vi "XY Graph Get Plot Name Format String.vi"(8 "error in (no error)":errorcluster, 11 "Select(T)/Deselect(F)":bool) -> (0 "error out":errorcluster, 1 "Cancelled?":bool, 3 "String Format":string)   [LabVIEW 2021, in "XY Graph Add-Ons.lvlib"]
doc: "Displays a standard dialog box that prompts users to enter information, such as a user name and password.\n--------------------\n\nThis Express VI is configured as follows:\n\nMessage to Display to the User:Select plot names matching the following format:\nThe inputs are: \nText Entry Box: String Format"
uses:
  XY Graph Add-Ons.lvlib
panel:
  in  "String Format":string
  out "String":string="Select plot names matching the following format:"
  in  "Cancel":bool
  in  "OK":bool caption="OK2"
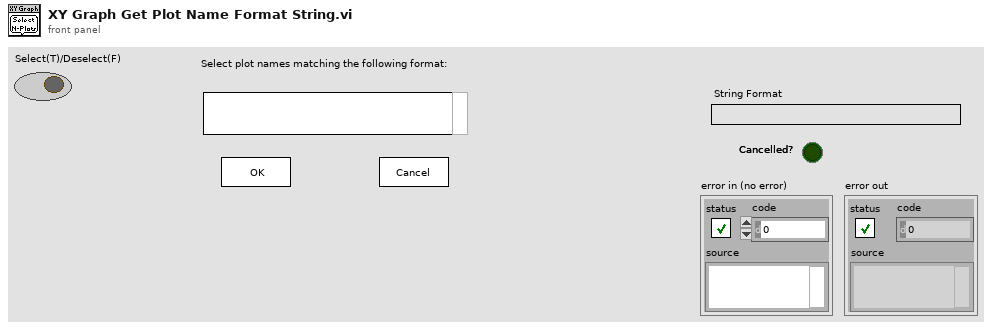
[diagram p1: front panel]
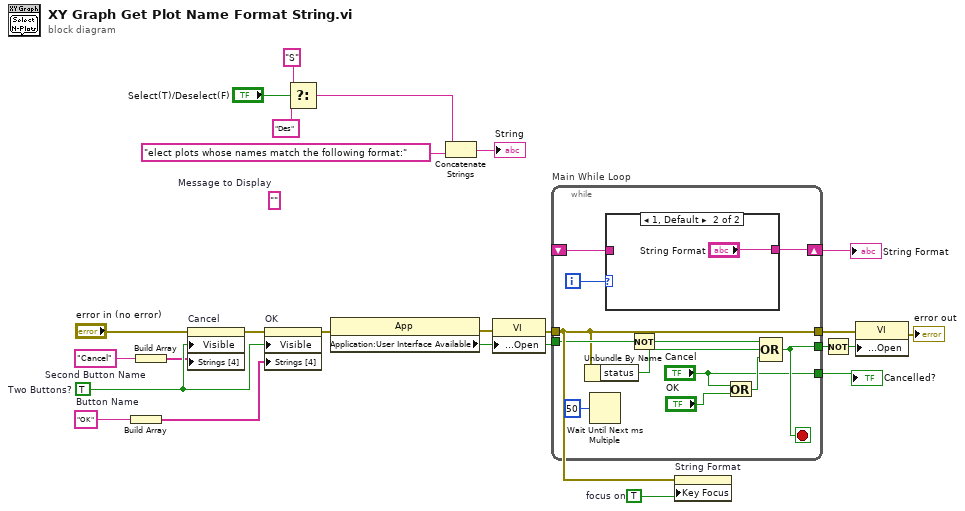
[diagram p0: block diagram]
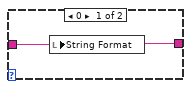
[diagram p2: hidden frame]
diagram:
  w11 = TRUE  # focus on
  w19 = "Cancel"  # Second Button Name
  w17 = "OK"  # Button Name
  (unwired) ""  # Message to Display
  w24 = TRUE  # Two Buttons?
  n1 = Build Array(w17) -> (w18:string[])
  n2 = Build Array(w19) -> (w20:string[])
  n3 = property on="Cancel" class="Bool"(error in="error in (no error)", "Visible"=w24, "Strings [4]"=w20) -> (error out=w23:errorcluster)  [unwired: 1 in, 1 out]
  n4 = property on="OK" class="Bool"(error in=w23, "Visible"=w24, "Strings [4]"=w18) -> (error out=w9:errorcluster)  [unwired: 1 in, 1 out]
  n5 = Select(t="S" ("string"), s="Select(T)/Deselect(F)", f="Des") -> (s? t:f=w3:string)
  n6 = property class="App"(error in=w9) -> (error out=w8:errorcluster, "Application:User Interface Available"=w12:bool)  [unwired: 1 in, 1 out]
  n7 = Concatenate Strings(w3, "elect plots whose names match the following format:" ("String")) -> (→"String":string)
  n8 = property class="VI"(error in=w8, "Front Panel Window:Open"=w12) -> (error out=w16:errorcluster)  [unwired: 1 in, 1 out]
  n9 = while "Main While Loop" {
    tunnel: w12 -> [w34]
    tunnel: [w32] -> w21
    tunnel: w16 -> [w31]
    tunnel: [w31] -> w14
    tunnel: ["Cancel"] -> w10
    shift-right: [w25] -> w1
    shift-left: _ -> [w26]
    i -> [w27]
    stop <- w32 stop-if-true
    n10 = Unbundle By Name(w31) -> ("status"=w29:bool)
    n11 = Wait Until Next ms Multiple(millisecond multiple=u32 50) -> ()  [unwired: 1 out]
    n12 = case shown="1, Default" w27 {
      tunnel: w26 -> [w37 _]
      tunnel: [w37 "String Format"] -> w25
      frame 0 {
        n13 = local write "String Format"(w37) -> ()
      }
      frame 1, Default {
      }
    }
    n14 = Not(x=w34) -> (.not. x?=w33:bool)
    n15 = Or(x="Cancel", y="OK") -> (x .or. y?=w30:bool)
    n16 = Compound Arithmetic op=OR(w33, w29, w30) -> (w32:bool)
  }
  "Cancelled?" <- w10
  "String Format" <- w1
  n17 = property on="String Format" class="Str"(error in=w16, "Key Focus"=w11) -> ()  [unwired: 1 in, 2 out]
  n18 = Not(x=w21) -> (.not. x?=w22:bool)
  n19 = property class="VI"(error in=w14, "Front Panel Window:Open"=w22) -> (error out=→"error out":errorcluster)  [unwired: 1 in, 1 out]
